vi "Compare Script Parameters.vi"(1 "Run Instance B":refnum<class "Run Instance.lvclass">, 2 "Run Instance A":refnum<class "Run Instance.lvclass">) -> (0 "Same?":bool)   [LabVIEW 2020, in "Run Utilities.lvlib"]
doc: "Compare the names of paramters used by the script. Vi returns true if the lists are the same"
uses:
  Run Utilities.lvlib
  Run Instance/Run Instance.lvclass
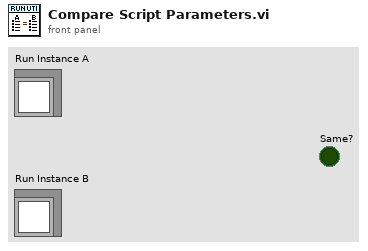
[diagram p1: front panel]
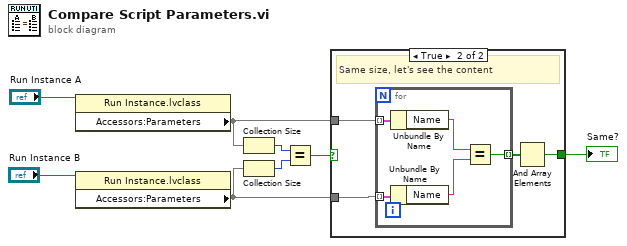
[diagram p0: block diagram]
diagram:
  n1 = property class="Run Instance.lvclass"(reference="Run Instance A") -> ("Accessors:Parameters"=w3:map{string, string})  [unwired: 1 in, 2 out]
  n2 = property class="Run Instance.lvclass"(reference="Run Instance B") -> ("Accessors:Parameters"=w2:map{string, string})  [unwired: 1 in, 2 out]
  n3 = Collection Size(1:w3) -> (0:w6:i32)
  n4 = Collection Size(1:w2) -> (0:w5:i32)
  n5 = Equal?(x=w6, y=w5) -> (x = y?=w4:bool)
  n6 = case shown="True" w4 {
    selector: w4 -> [w9 _]
    tunnel: w3 -> [_ w13]
    tunnel: w2 -> [_ w12]
    tunnel: [w9 w10] -> w1
    frame False {
      # "Different size of the list of parameters, therefore, they are different instances"
    }
    frame True {
      # "Same size, let's see the content"
      n7 = for {
        tunnel: w13 -> [w18] mode=indexing
        tunnel: w12 -> [w17] mode=indexing
        tunnel: [w14] -> w11 mode=indexing
        n8 = Unbundle By Name(w18) -> ("Name"=w16:string)
        n9 = Unbundle By Name(w17) -> ("Name"=w15:string)
        n10 = Equal?(x=w16, y=w15) -> (x = y?=w14:bool)
      }
      n11 = And Array Elements(Boolean array=w11) -> (logical AND=w10:bool)
    }
  }
  "Same?" <- w1
